vi "Voltages1.1.vi"(10 "delay before read (ms)":u32=500, 11 "VISA PS":refnum<visa-resource-name>="COM1") -> ()   [LabVIEW 2013]
panel:
  out "appended array":dbl[](array[numeric])
  in  "VISA Scope":refnum<visa-resource-name>="COM1"
  out "Array of Voltages":string[](array[string])
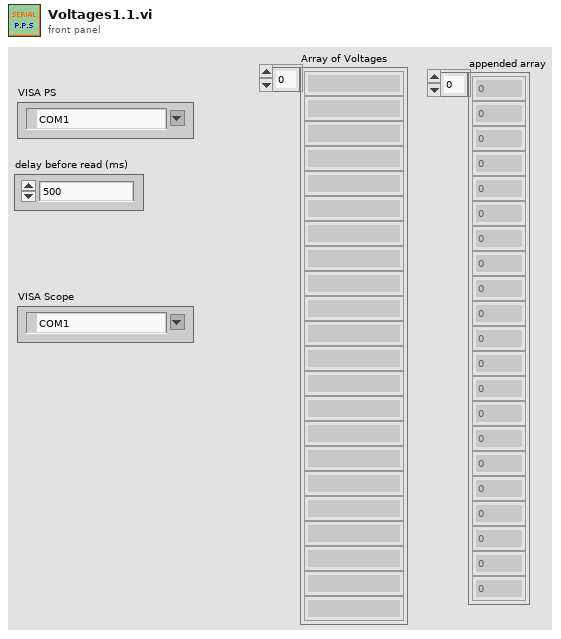
[diagram p1: front panel]
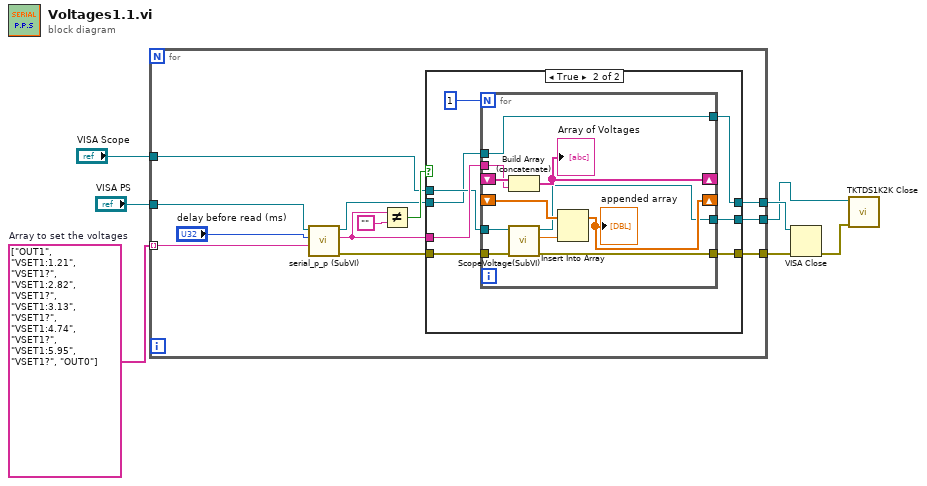
[diagram p0: block diagram]
diagram:
  w5 = string[] ["OUT1", "VSET1:1.21", "VSET1?", "VSET1:2.82", "VSET1?", "VSET1:3.13", "VSET1?", "VSET1:4.74", "VSET1?", "VSET1:5.95", "VSET1?", "OUT0"]  # Array to set the voltages
  n1 = for {
    tunnel: "VISA PS" -> [w18]
    tunnel: w5 -> [w17] mode=indexing
    tunnel: [w9] -> w6
    tunnel: "VISA Scope" -> [w13]
    tunnel: [w11] -> w3
    tunnel: [w8] -> w2
    n2 = call "serial_p_p (SubVI).vi"("Command"=w17, "delay before read (ms)"="delay before read (ms)", "VISA Refnum in"=w18) -> ("error out"=w12:errorcluster, "read buffer"=w14:string, "VISA Refnum out"=w10:refnum<visa-resource-name>)  [unwired: 6 in]
    n3 = Not Equal?(x=w14, y="") -> (x != y?=w16:bool)
    n4 = case shown="True" w16 {
      tunnel: w14 -> [_ w30]
      tunnel: w13 -> [w21 w28]
      tunnel: w12 -> [w22 w27]
      tunnel: [w22 w25] -> w11
      tunnel: [w21 w26] -> w8
      tunnel: w10 -> [w20 w24]
      tunnel: [w20 w23] -> w9
      frame False {
      }
      frame True {
        n5 = for {
          N: 1 -> [_]
          tunnel: w30 -> [w39]
          shift-right: [w41] -> _
          shift-left: _ -> [w40]
          tunnel: w28 -> [w36]
          shift-right: [w37] -> _
          shift-left: _ -> [w38]
          tunnel: w27 -> [w31]
          tunnel: [w34] -> w26
          tunnel: [w33] -> w25
          tunnel: w24 -> [w32]
          tunnel: [w32] -> w23
          n6 = Build Array (concatenate)(w40, w39) -> (w41:string[])
          "Array of Voltages" <- w41
          n7 = call "ScopeVoltage(SubVI).vi"("error in (no error)"=w31, "VISA Refnum in"=w36) -> ("error out"=w33:errorcluster, "Measurement"=w35:dbl, "VISA Refnum out"=w34:refnum<visa-resource-name>)  [unwired: 6 in, 1 out]
          n8 = Insert Into Array(array=w38, new element=w35) -> (w37:dbl[])  [unwired: 1 in]
          "appended array" <- w37
        }
      }
    }
  }
  n9 = VISA Close(VISA resource name=w6, error in (no error)=w3) -> (error out=w1:errorcluster)
  n10 = call <instrlib>:"TKTDS1K2K Close.vi"("error in (no error)"=w1, "VISA session"=w2) -> ()  [unwired: 9 in, 1 out]
